vi "GetSyringeXYZ.vi"(8 "error in":errorcluster, 10 "Position":enum16{"1", "2"}(ring), 11 "Zone":enum16{"ZoneA", "ZoneB", "ZoneC", "ZoneD"}(ring)) -> (0 "Error out":errorcluster, 1 "SyringeZ":dbl=87.501, 2 "SyringeY":dbl format="%#_7g", 3 "SyringeX":dbl format="%#_7g")   [LabVIEW 2019]
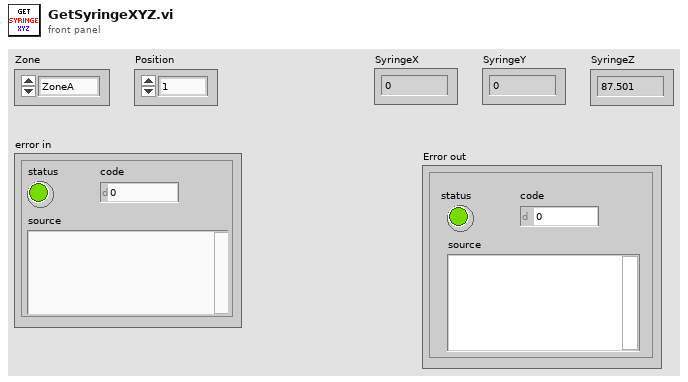
[diagram p1: front panel]
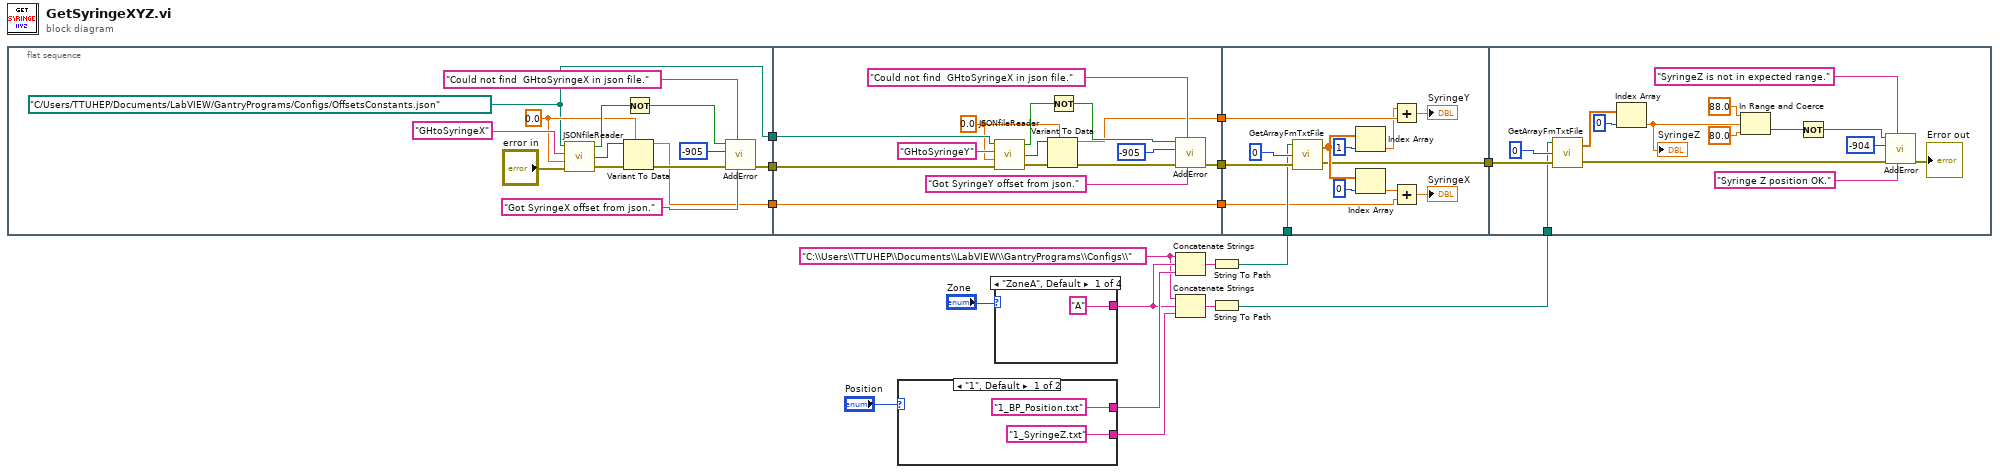
[diagram p0: block diagram]
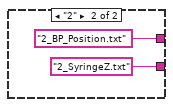
[diagram p2: hidden frame]
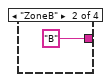
[diagram p3: hidden frame]
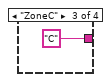
[diagram p4: hidden frame]
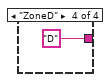
[diagram p5: hidden frame]
diagram:
  w2 = "C:\\Users\\TTUHEP\\Documents\\LabVIEW\\GantryPrograms\\Configs\\"
  n1 = flat-sequence {
    tunnel: [w26] -> w15
    tunnel: [w20] -> w14
    tunnel: [w19] -> w13
    tunnel: w15 -> [w37]
    tunnel: w14 -> [w38]
    tunnel: w13 -> [w46]
    tunnel: [w46] -> w12
    tunnel: [w36] -> w11
    tunnel: [w35] -> w10
    tunnel: w12 -> [w47]
    tunnel: w11 -> [w56]
    tunnel: w10 -> [w51]
    tunnel: w9 -> [w54]
    tunnel: [w53] -> w8
    tunnel: w8 -> [w74]
    tunnel: w7 -> [w72]
    frame #0 {
      w26 = path "C:/Users/TTUHEP/Documents/LabVIEW/GantryPrograms/Configs/OffsetsConstants.json" ("OffsetsConstantsForSyringeXY")
      w29 = 0.0
      n2 = call "JSONfileReader.vi"("error in"="error in", "Variant"=w29, "ItemName"="GHtoSyringeX", "FileIn"=w26) -> ("error out"=w27:errorcluster, "Data"=w28:variant, "Found"=w30:bool)
      n3 = Variant To Data(error in=w27, type=w29, Variant=w28) -> (data=w19:dbl, error out=w25:errorcluster)
      n4 = Not(x=w30) -> (.not. x?=w24:bool)
      n5 = call "AddError.vi"("NoErrorMessage"="Got SyringeX offset from json.", "ErrorMessage"="Could not find  GHtoSyringeX in json file.", "error in"=w25, "code"=-905, "Error?"=w24) -> ("Error out"=w20:errorcluster)  [unwired: 6 in]
    }
    frame #1 {
      w32 = 0.0
      n6 = call "JSONfileReader.vi"("error in"=w38, "Variant"=w32, "ItemName"="GHtoSyringeY", "FileIn"=w37) -> ("error out"=w43:errorcluster, "Data"=w42:variant, "Found"=w41:bool)
      n7 = Variant To Data(error in=w43, type=w32, Variant=w42) -> (data=w35:dbl, error out=w44:errorcluster)
      n8 = Not(x=w41) -> (.not. x?=w45:bool)
      n9 = call "AddError.vi"("NoErrorMessage"="Got SyringeY offset from json.", "ErrorMessage"="Could not find  GHtoSyringeX in json file.", "error in"=w44, "code"=-905, "Error?"=w45) -> ("Error out"=w36:errorcluster)  [unwired: 6 in]
    }
    frame #2 {
      n10 = call "GetArrayFmTxtFile.vi"("error in"=w56, "LineNo."=0, "TextFile"=w54) -> ("error out"=w53:errorcluster, "Array"=w59:dbl[])
      n11 = Index Array(array=w59, index=1) -> (element=w50:dbl)
      n12 = Index Array(array=w59, index=0) -> (element=w52:dbl)
      n13 = Add(x=w50, y=w51) -> (x+y=→"SyringeY":dbl)
      n14 = Add(x=w52, y=w47) -> (x+y=→"SyringeX":dbl)
    }
    frame #3 {
      n15 = call "GetArrayFmTxtFile.vi"("error in"=w74, "LineNo."=0, "TextFile"=w72) -> ("error out"=w66:errorcluster, "Array"=w62:dbl[])
      n16 = Index Array(array=w62, index=0) -> (element=w69:dbl)
      "SyringeZ" <- w69
      n17 = In Range and Coerce(upper limit=88.0, x=w69, lower limit=80.0) -> (In Range?=w70:bool)  [unwired: 1 out]
      n18 = Not(x=w70) -> (.not. x?=w71:bool)
      n19 = call "AddError.vi"("NoErrorMessage"="Syringe Z position OK.", "ErrorMessage"="SyringeZ is not in expected range.", "error in"=w66, "code"=-904, "Error?"=w71) -> ("Error out"=→"Error out":errorcluster)  [unwired: 6 in]
    }
  }
  n20 = case shown="\"1\", Default" "Position" {
    tunnel: ["1_SyringeZ.txt" ("string") "2_SyringeZ.txt" ("string")] -> w4
    tunnel: ["1_BP_Position.txt" "2_BP_Position.txt"] -> w6
    frame "1", Default {
    }
    frame "2" {
    }
  }
  n21 = case shown="\"ZoneA\", Default" "Zone" {
    tunnel: ["A" "B" "C" "D"] -> w5
    frame "ZoneA", Default {
    }
    frame "ZoneB" {
    }
    frame "ZoneC" {
    }
    frame "ZoneD" {
    }
  }
  n22 = Concatenate Strings(w2, w5, w6) -> (w1:string)
  n23 = Concatenate Strings(w2, w5, w4) -> (w3:string)
  n24 = String To Path(string=w1) -> (path=w9:path)
  n25 = String To Path(string=w3) -> (path=w7:path)
